vi "Test.vi"() -> ()   [LabVIEW 2015, in "HMI Messages.lvclass"]
uses:
  HMI Messages.lvclass
  HMI Messages.lvclass/HMI Messages.ctl
  Re-use Libraries/Utility/Utility.lvlib
panel:
  out "Array":string[](array[string])
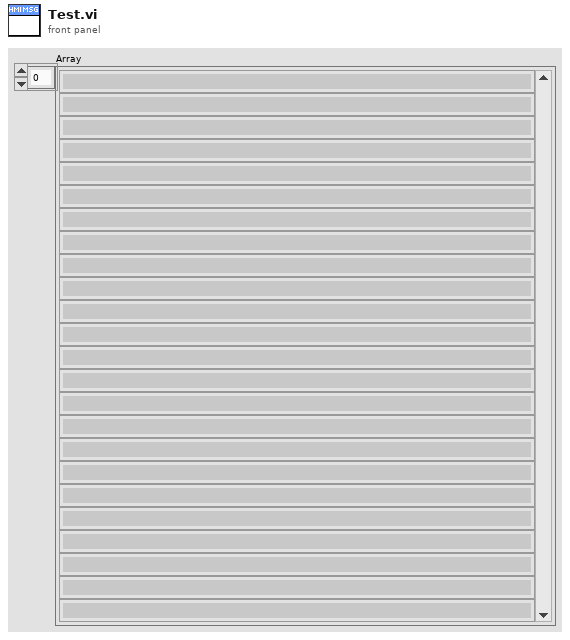
[diagram p1: front panel]
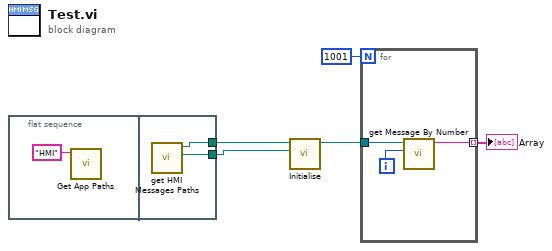
[diagram p0: block diagram]
diagram:
  n1 = flat-sequence {
    tunnel: [w8] -> w2
    tunnel: [w7] -> w1
    frame #0 {
      n2 = call "Get App Paths.vi"("Build Name"="HMI") -> ()  [unwired: 9 in, 2 out]
    }
    frame #1 {
      n3 = call "get HMI Messages Paths.vi"() -> ("PC Messages"=w7:path, "PLC Messages"=w8:path)  [unwired: 10 in]
    }
  }
  n4 = call "Initialise.vi"("PC Messages Definitions File"=w1, "PLC Messages Definitions File"=w2) -> ("HMI Messages out"=w5:refnum<class "HMI Messages.lvclass">)  [unwired: 8 in, 1 out]
  n5 = for {
    N: 1001 -> [_]
    tunnel: w5 -> [w11]
    tunnel: [w9] -> w3 mode=indexing
    i -> [w10]
    n6 = call "get Message By Number.vi"("Message Number"=w10, "HMI Messages in"=w11) -> ("Message"=w9:string)  [unwired: 9 in]
  }
  "Array" <- w3
